vi "Clean Duplicate Engine Mapping.vi"(7 "modules":T2[](array[typedef]), 8 "error in (no error)":errorcluster, 9 "New Children":T1[](array[typedef]), 10 "Old Children":T1[](array[typedef]), 11 "Engine configuration in":refnum<class "NISE_CEF_serializable configuration.lvclass">) -> (0 "error out":errorcluster, 3 "Engine configuration out":refnum<class "NISE_CEF_serializable configuration.lvclass">)   [LabVIEW 2013, in "Standard Editor.lvlib"]
uses:
  Standard Editor.lvlib
  <vilib>/NI/Configuration Framework/serializable configuration/NISE_CEF_serializable configuration.lvclass
  Framework Configuration Classes/class cache/class metadata.ctl
  <vilib>/NI/Tag Bus Module Framework/root configuration/Target Types.ctl
  <vilib>/NI/Configuration Framework/Node/NodeRef.ctl
  <vilib>/NI/Configuration Framework/Node/NISE_CEF_Node.lvclass
  <vilib>/NI/Configuration Framework/serializable node/NISE_CEF_serializable node.lvclass
  <vilib>/NI/Module Execution Interface/Engine Configuration/engine configuration.lvclass
  <vilib>/NI/Configuration Framework/serializable configuration/NISE_CEF_serializable configuration.lvclass/NISE_CEF_serializable configuration.ctl
  <vilib>/NI/Configuration Framework/serializable configuration/Read UID.vi
  <vilib>/Utility/LVClass/Get LV Class Name.vi
  <vilib>/NI/Configuration Framework/error generator/NISE_error generator.vi
  <vilib>/NI/Tag Bus Module Framework/root configuration/TBM configuration.lvclass
  Framework Configuration Classes/class cache/PL_class cache.lvlib
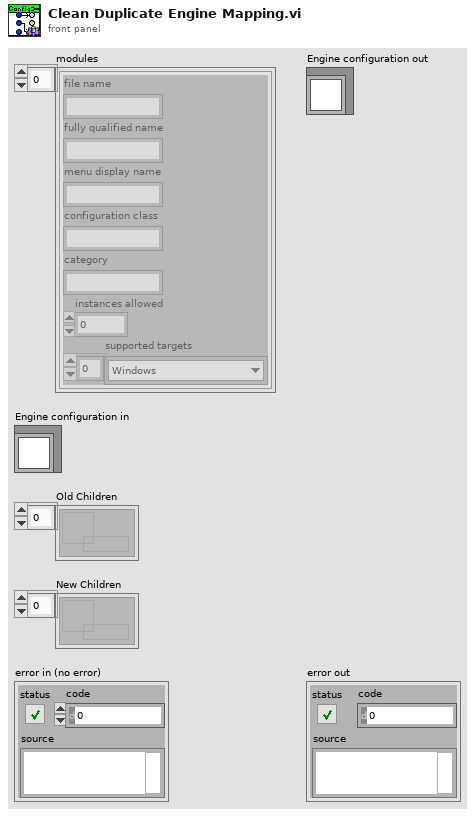
[diagram p1: front panel]
types:
  T1 = typedef "NISE_CEF_Node.lvclass/NodeRef.ctl" = refnum<data-value>
  T2 = typedef "PL_class cache.lvlib/class metadata.ctl" = cluster{"file name":string, "fully qualified name":string, "menu display name":string, "configuration class":string, "category":string, "instances allowed":i32, "supported targets":T3[]}
  T3 = typedef "TBM configuration.lvclass/Target Types.ctl" = enum16{"Windows", "Mac", "Linux", "Linux RT ARM", "VxWorks", "Pharlap", "Other", "Linux RT x64"}
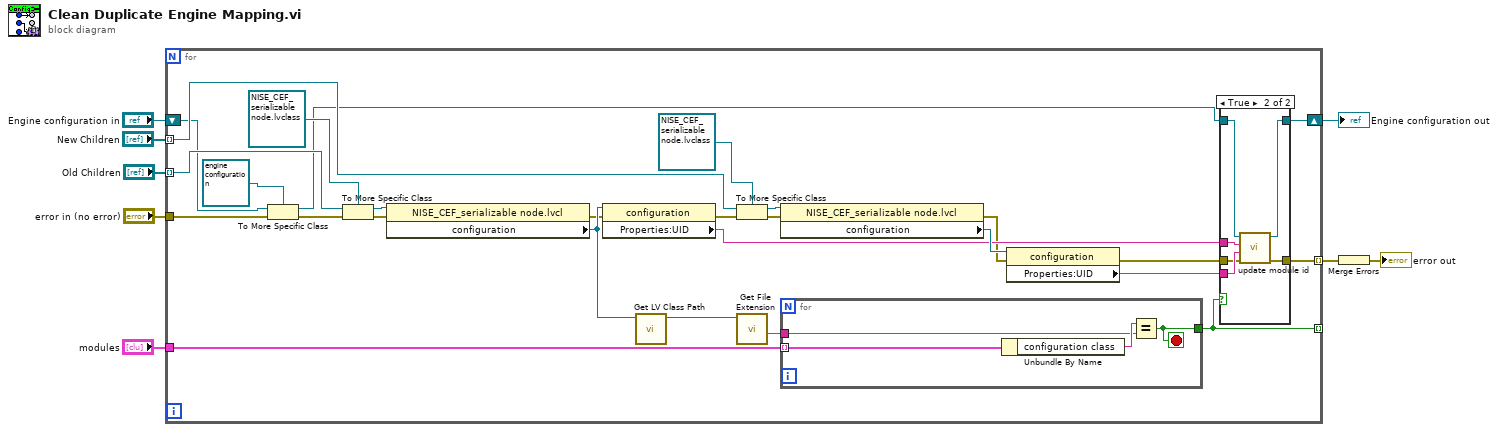
[diagram p0: block diagram]
diagram:
  n1 = for {
    tunnel: "New Children" -> [w35] mode=indexing
    tunnel: "Old Children" -> [w34] mode=indexing
    tunnel: "modules" -> [w27]
    tunnel: [w9] -> _ mode=indexing
    shift-right: [w19] -> w5
    shift-left: "Engine configuration in" -> [w22]
    tunnel: "error in (no error)" -> [w17]
    tunnel: [w18] -> w7 mode=indexing
    n2 = To More Specific Class(target class=refnum<class "engine configuration.lvclass"> refnum ("engine configuration in"), reference=w22, error in=w17) -> (specific class reference=w21:refnum<class "engine configuration.lvclass">, error out=w16:errorcluster)
    n3 = To More Specific Class(target class=refnum<data-value> refnum, reference=w34, error in=w16) -> (specific class reference=w30:refnum<data-value>, error out=w15:errorcluster)
    n4 = property class="NISE_CEF_serializable node.lvcl"(reference=w30, error in=w15) -> (error out=w14:errorcluster, "configuration"=w26:refnum<class "NISE_CEF_serializable configuration.lvclass">)  [unwired: 1 out]
    n5 = property class="configuration"(reference=w26, error in=w14) -> (error out=w13:errorcluster, "Properties:UID"=w23:string)  [unwired: 1 out]
    n6 = call <vilib>:"Get LV Class Path.vi"("object"=w26) -> ("class path"=w29:path)  [unwired: 9 in, 1 out]
    n7 = To More Specific Class(target class=refnum<data-value> refnum, reference=w35, error in=w13) -> (specific class reference=w31:refnum<data-value>, error out=w12:errorcluster)
    n8 = call <vilib>:"Get File Extension.vi"("file"=w29) -> ("filename without extension"=w28:string)  [unwired: 7 in, 3 out]
    n9 = property class="NISE_CEF_serializable node.lvcl"(reference=w31, error in=w12) -> (error out=w11:errorcluster, "configuration"=w25:refnum<class "NISE_CEF_serializable configuration.lvclass">)  [unwired: 1 out]
    n10 = for {
      tunnel: w27 -> [w46] mode=indexing
      tunnel: w28 -> [w44]
      tunnel: [w43] -> w9
      stop <- w43 stop-if-true
      n11 = Unbundle By Name(w46) -> ("configuration class"=w45:string)
      n12 = Equal?(x=w45, y=w44) -> (x = y?=w43:bool)
    }
    n13 = property class="configuration"(reference=w25, error in=w11) -> (error out=w10:errorcluster, "Properties:UID"=w24:string)  [unwired: 1 out]
    n14 = case shown="True" w9 {
      tunnel: w24 -> [_ w41]
      tunnel: w23 -> [_ w42]
      tunnel: w21 -> [w36 w40]
      tunnel: [w36 w39] -> w19
      tunnel: [_ w38] -> w18
      tunnel: w10 -> [_ w37]
      frame False {
      }
      frame True {
        n15 = call <vilib>:"update module id.vi"("error in (no error)"=w37, "New Id"=w41, "Old Id"=w42, "engine configuration in"=w40) -> ("error out"=w38:errorcluster, "engine configuration out"=w39:refnum<class "engine configuration.lvclass">)  [unwired: 6 in]
      }
    }
  }
  "Engine configuration out" <- w5
  n16 = Merge Errors(w7) -> (→"error out":errorcluster)
